vi "MP6_micro_pump.vi"() -> ()   [LabVIEW 2024]
uses:
  <vilib>/Instr/_visa.llb/VISA Configure Serial Port (Instr).vi
panel:
  out "P2V_output":string
  in  "P2V?":bool
  in  "Continuos V":bool
  out "P1V_output":string
  in  "P1V?":bool
  in  "P2V_value":u8
  in  "P2V_set":bool
  in  "F1_value":u8=100
  in  "F1_set":bool
  in  "P1V_value":u8=200
  in  "P1V_set":bool
  out "Output":string="150\r\n"
  in  "Input":string="P5V?\r\n"
  in  "Send Command":bool
  in  "P2OFF":bool
  in  "P2ON":bool
  in  "P1OFF":bool
  in  "P1ON":bool
  out "error out":errorcluster={"status"=FALSE, "code"=1073676294, "source"="VISA Read in MP6_micro_pump.vi"}
  in  "VISA resource name":refnum<visa-resource-name>="COM3"
  in  "Close connection":bool
  in  "Open connection":bool
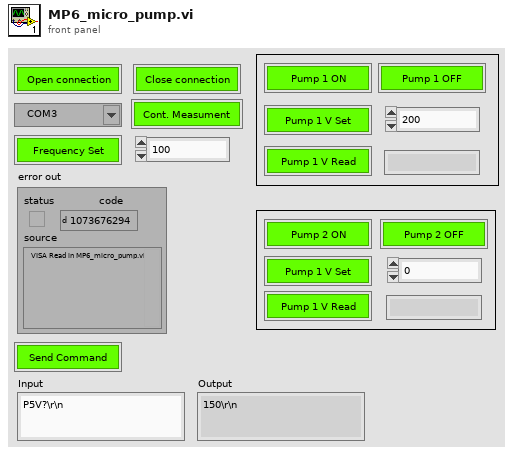
[diagram p1: front panel]
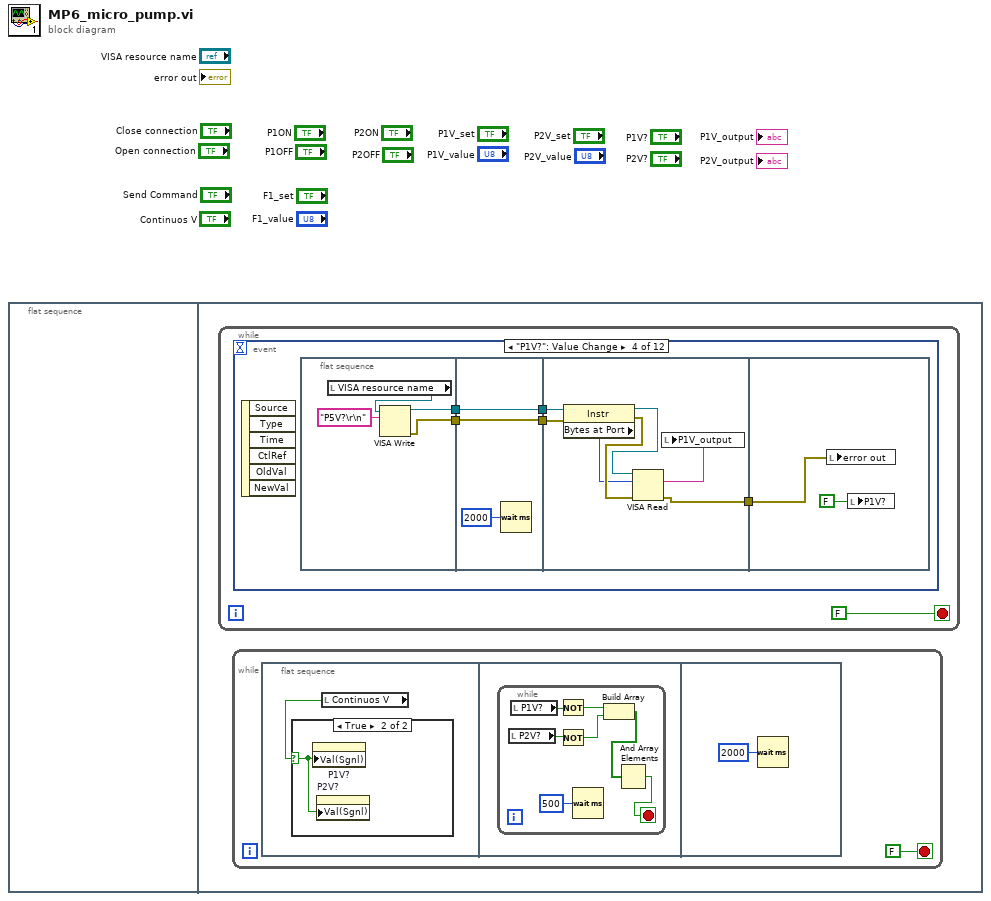
[diagram p0: block diagram]
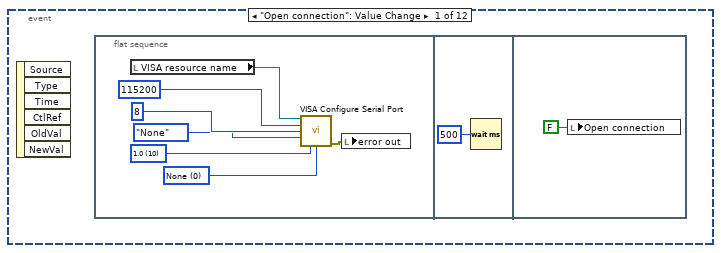
[diagram p3: hidden frame]
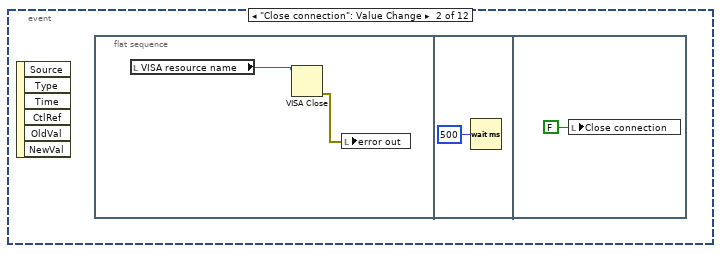
[diagram p4: hidden frame]
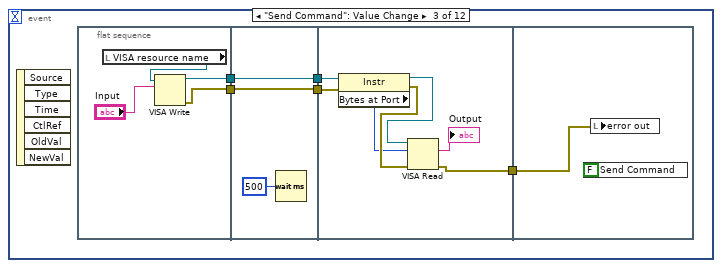
[diagram p5: hidden frame]
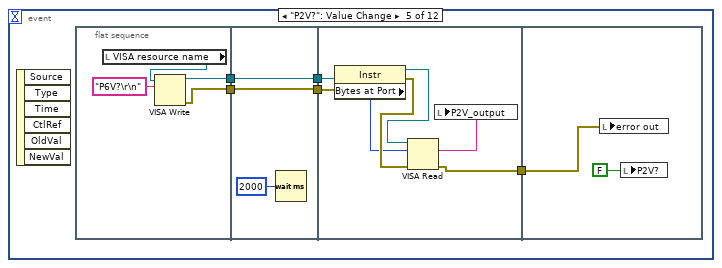
[diagram p6: hidden frame]
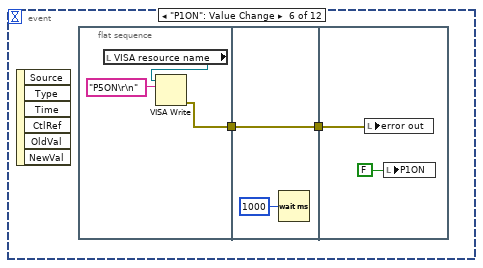
[diagram p7: hidden frame]
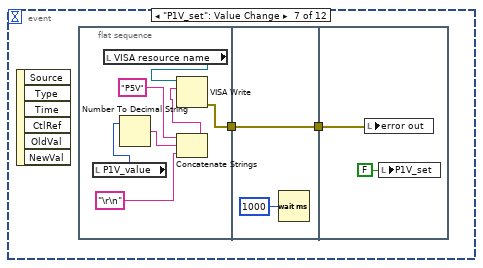
[diagram p8: hidden frame]
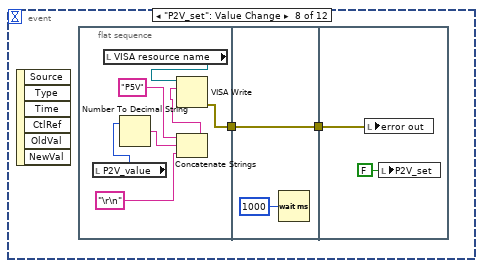
[diagram p9: hidden frame]
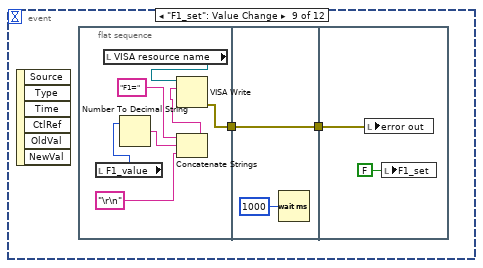
[diagram p10: hidden frame]
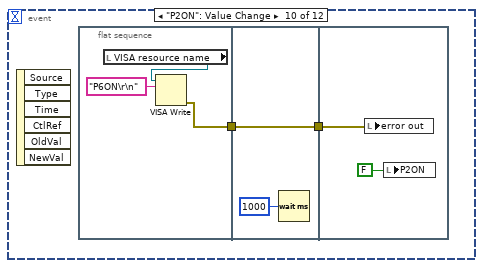
[diagram p11: hidden frame]
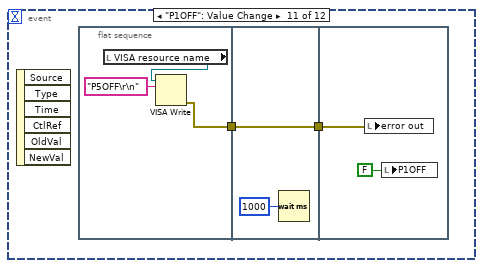
[diagram p12: hidden frame]
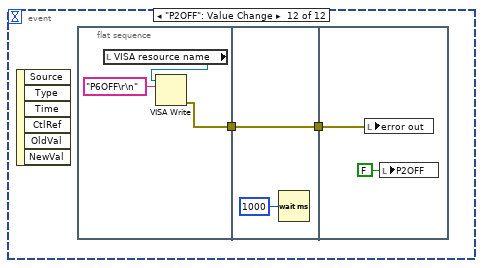
[diagram p13: hidden frame]
diagram:
  n1 = flat-sequence {
    frame #0 {
    }
    frame #1 {
      n2 = while {
        stop <- FALSE stop-if-true
        n3 = event shown="[3] \"P1V?\": Value Change" {
          selector: _ -> [_ _ _ _ _ _ _ _ _ _ _ _]
          dyn-events: _ -> [_ _ _ _ _ _ _ _ _ _ _ _]
          timeout: _ -> [_ _ _ _ _ _ _ _ _ _ _ _]
          event "Open connection": Value Change {
            n4 = event-data() -> ()  [unwired: 1 in, 6 out]
            n5 = flat-sequence {
              frame #0 {
                w15 = u16 0 items=["None", "XON/XOFF", "RTS/CTS", "XON/XOFF & RTS/CTS", "DTR/DSR", "XON/XOFF & DTR/DSR"] ("flow control (0:none)")
                w16 = u16 10 items=["1.0"=10, "1.5"=15, "2.0"=20] ("stop bits (10: 1 bit)")
                n6 = local read "VISA resource name"() -> (w13:refnum<visa-resource-name>)
                n7 = call-poly "VISA Configure Serial Port"("VISA resource name"=w13, "baud rate (9600)"=u32 115200, "data bits (8)"=u16 8, "parity (0:none)"=enum16{"None", "Odd", "Even", "Mark", "Space"}."None", "stop bits (10: 1 bit)"=w16, "flow control (0:none)"=w15) -> ("error out"=w14:errorcluster)  [unwired: 8 in, 1 out]
                n8 = local write "error out"(w14) -> ()
              }
              frame #1 {
                n9 = Wait (ms)(milliseconds to wait=u32 500) -> ()  [unwired: 1 out]
              }
              frame #2 {
                n10 = local write "Open connection"(FALSE ("Open connection")) -> ()
              }
            }
          }
          event "Close connection": Value Change {
            n11 = event-data() -> ()  [unwired: 1 in, 6 out]
            n12 = flat-sequence {
              frame #0 {
                n13 = local read "VISA resource name"() -> (w23:refnum<visa-resource-name>)
                n14 = VISA Close(VISA resource name=w23) -> (error out=w22:errorcluster)  [unwired: 1 in]
                n15 = local write "error out"(w22) -> ()
              }
              frame #1 {
                n16 = Wait (ms)(milliseconds to wait=u32 500) -> ()  [unwired: 1 out]
              }
              frame #2 {
                n17 = local write "Close connection"(FALSE ("Open connection")) -> ()
              }
            }
          }
          event "Send Command": Value Change {
            n18 = event-data() -> ()  [unwired: 1 in, 6 out]
            n19 = flat-sequence {
              tunnel: [w33] -> w29
              tunnel: [w31] -> w26
              tunnel: [w37] -> w30
              tunnel: w29 -> [w37]
              tunnel: [w36] -> w27
              tunnel: w26 -> [w36]
              tunnel: w30 -> [w43]
              tunnel: [w39] -> w28
              tunnel: w27 -> [w44]
              tunnel: w28 -> [w46]
              frame #0 {
                n20 = local read "VISA resource name"() -> (w34:refnum<visa-resource-name>)
                n21 = VISA Write(VISA resource name=w34, write buffer="Input") -> (VISA resource name out=w31:refnum<visa-resource-name>, error out=w33:errorcluster)  [unwired: 1 in, 1 out]
              }
              frame #1 {
                n22 = Wait (ms)(milliseconds to wait=u32 500) -> ()  [unwired: 1 out]
              }
              frame #2 {
                n23 = property class="Instr"(reference=w44, error in=w43) -> (reference out=w41:refnum<visa-resource-name>, error out=w42:errorcluster, "Bytes at Port"=w40:u32)
                n24 = VISA Read(VISA resource name=w41, byte count=w40, error in (no error)=w42) -> (read buffer=→"Output":string, error out=w39:errorcluster)  [unwired: 2 out]
              }
              frame #3 {
                n25 = local write "Send Command"(FALSE ("P1OFF")) -> ()
                n26 = local write "error out"(w46) -> ()
              }
            }
          }
          event "P1V?": Value Change {
            n27 = event-data() -> ()  [unwired: 1 in, 6 out]
            n28 = flat-sequence {
              tunnel: [w54] -> w50
              tunnel: [w53] -> w47
              tunnel: [w58] -> w51
              tunnel: w50 -> [w58]
              tunnel: [w57] -> w48
              tunnel: w47 -> [w57]
              tunnel: w51 -> [w64]
              tunnel: [w60] -> w49
              tunnel: w48 -> [w65]
              tunnel: w49 -> [w67]
              frame #0 {
                n29 = local read "VISA resource name"() -> (w55:refnum<visa-resource-name>)
                n30 = VISA Write(VISA resource name=w55, write buffer="P5V?\r\n") -> (VISA resource name out=w53:refnum<visa-resource-name>, error out=w54:errorcluster)  [unwired: 1 in, 1 out]
              }
              frame #1 {
                n31 = Wait (ms)(milliseconds to wait=u32 2000) -> ()  [unwired: 1 out]
              }
              frame #2 {
                n32 = property class="Instr"(reference=w65, error in=w64) -> (reference out=w62:refnum<visa-resource-name>, error out=w63:errorcluster, "Bytes at Port"=w61:u32)
                n33 = VISA Read(VISA resource name=w62, byte count=w61, error in (no error)=w63) -> (read buffer=w59:string, error out=w60:errorcluster)  [unwired: 2 out]
                n34 = local write "P1V_output"(w59) -> ()
              }
              frame #3 {
                n35 = local write "error out"(w67) -> ()
                n36 = local write "P1V?"(FALSE ("P1OFF")) -> ()
              }
            }
          }
          event "P2V?": Value Change {
            n37 = event-data() -> ()  [unwired: 1 in, 6 out]
            n38 = flat-sequence {
              tunnel: [w75] -> w71
              tunnel: [w74] -> w68
              tunnel: [w79] -> w72
              tunnel: w71 -> [w79]
              tunnel: [w78] -> w69
              tunnel: w68 -> [w78]
              tunnel: w72 -> [w85]
              tunnel: [w81] -> w70
              tunnel: w69 -> [w86]
              tunnel: w70 -> [w88]
              frame #0 {
                n39 = local read "VISA resource name"() -> (w76:refnum<visa-resource-name>)
                n40 = VISA Write(VISA resource name=w76, write buffer="P6V?\r\n") -> (VISA resource name out=w74:refnum<visa-resource-name>, error out=w75:errorcluster)  [unwired: 1 in, 1 out]
              }
              frame #1 {
                n41 = Wait (ms)(milliseconds to wait=u32 2000) -> ()  [unwired: 1 out]
              }
              frame #2 {
                n42 = property class="Instr"(reference=w86, error in=w85) -> (reference out=w83:refnum<visa-resource-name>, error out=w84:errorcluster, "Bytes at Port"=w82:u32)
                n43 = VISA Read(VISA resource name=w83, byte count=w82, error in (no error)=w84) -> (read buffer=w80:string, error out=w81:errorcluster)  [unwired: 2 out]
                n44 = local write "P2V_output"(w80) -> ()
              }
              frame #3 {
                n45 = local write "error out"(w88) -> ()
                n46 = local write "P2V?"(FALSE ("P1OFF")) -> ()
              }
            }
          }
          event "P1ON": Value Change {
            n47 = event-data() -> ()  [unwired: 1 in, 6 out]
            n48 = flat-sequence {
              tunnel: [w91] -> w89
              tunnel: [w94] -> w90
              tunnel: w89 -> [w94]
              tunnel: w90 -> [w96]
              frame #0 {
                n49 = local read "VISA resource name"() -> (w93:refnum<visa-resource-name>)
                n50 = VISA Write(VISA resource name=w93, write buffer="P5ON\r\n") -> (error out=w91:errorcluster)  [unwired: 1 in, 2 out]
              }
              frame #1 {
                n51 = Wait (ms)(milliseconds to wait=u32 1000) -> ()  [unwired: 1 out]
              }
              frame #2 {
                n52 = local write "error out"(w96) -> ()
                n53 = local write "P1ON"(FALSE ("P1OFF")) -> ()
              }
            }
          }
          event "P1V_set": Value Change {
            n54 = event-data() -> ()  [unwired: 1 in, 6 out]
            n55 = flat-sequence {
              tunnel: [w105] -> w98
              tunnel: [w107] -> w99
              tunnel: w98 -> [w107]
              tunnel: w99 -> [w109]
              frame #0 {
                n56 = local read "P1V_value"() -> (w104:u8)
                n57 = local read "VISA resource name"() -> (w106:refnum<visa-resource-name>)
                n58 = Number To Decimal String(number=w104) -> (decimal integer string=w103:string)  [unwired: 1 in]
                n59 = Concatenate Strings("P5V" ("write buffer"), w103, "\r\n" ("write buffer")) -> (w100:string)
                n60 = VISA Write(VISA resource name=w106, write buffer=w100) -> (error out=w105:errorcluster)  [unwired: 1 in, 2 out]
              }
              frame #1 {
                n61 = Wait (ms)(milliseconds to wait=u32 1000) -> ()  [unwired: 1 out]
              }
              frame #2 {
                n62 = local write "error out"(w109) -> ()
                n63 = local write "P1V_set"(FALSE ("P1OFF")) -> ()
              }
            }
          }
          event "P2V_set": Value Change {
            n64 = event-data() -> ()  [unwired: 1 in, 6 out]
            n65 = flat-sequence {
              tunnel: [w118] -> w111
              tunnel: [w120] -> w112
              tunnel: w111 -> [w120]
              tunnel: w112 -> [w122]
              frame #0 {
                n66 = local read "P2V_value"() -> (w117:u8)
                n67 = local read "VISA resource name"() -> (w119:refnum<visa-resource-name>)
                n68 = Number To Decimal String(number=w117) -> (decimal integer string=w116:string)  [unwired: 1 in]
                n69 = Concatenate Strings("P5V" ("write buffer"), w116, "\r\n" ("write buffer")) -> (w113:string)
                n70 = VISA Write(VISA resource name=w119, write buffer=w113) -> (error out=w118:errorcluster)  [unwired: 1 in, 2 out]
              }
              frame #1 {
                n71 = Wait (ms)(milliseconds to wait=u32 1000) -> ()  [unwired: 1 out]
              }
              frame #2 {
                n72 = local write "error out"(w122) -> ()
                n73 = local write "P2V_set"(FALSE ("P1OFF")) -> ()
              }
            }
          }
          event "F1_set": Value Change {
            n74 = event-data() -> ()  [unwired: 1 in, 6 out]
            n75 = flat-sequence {
              tunnel: [w131] -> w124
              tunnel: [w133] -> w125
              tunnel: w124 -> [w133]
              tunnel: w125 -> [w135]
              frame #0 {
                n76 = local read "F1_value"() -> (w130:u8)
                n77 = local read "VISA resource name"() -> (w132:refnum<visa-resource-name>)
                n78 = Number To Decimal String(number=w130) -> (decimal integer string=w129:string)  [unwired: 1 in]
                n79 = Concatenate Strings("F1=" ("write buffer"), w129, "\r\n" ("write buffer")) -> (w126:string)
                n80 = VISA Write(VISA resource name=w132, write buffer=w126) -> (error out=w131:errorcluster)  [unwired: 1 in, 2 out]
              }
              frame #1 {
                n81 = Wait (ms)(milliseconds to wait=u32 1000) -> ()  [unwired: 1 out]
              }
              frame #2 {
                n82 = local write "error out"(w135) -> ()
                n83 = local write "F1_set"(FALSE ("P1OFF")) -> ()
              }
            }
          }
          event "P2ON": Value Change {
            n84 = event-data() -> ()  [unwired: 1 in, 6 out]
            n85 = flat-sequence {
              tunnel: [w139] -> w137
              tunnel: [w142] -> w138
              tunnel: w137 -> [w142]
              tunnel: w138 -> [w144]
              frame #0 {
                n86 = local read "VISA resource name"() -> (w141:refnum<visa-resource-name>)
                n87 = VISA Write(VISA resource name=w141, write buffer="P6ON\r\n") -> (error out=w139:errorcluster)  [unwired: 1 in, 2 out]
              }
              frame #1 {
                n88 = Wait (ms)(milliseconds to wait=u32 1000) -> ()  [unwired: 1 out]
              }
              frame #2 {
                n89 = local write "error out"(w144) -> ()
                n90 = local write "P2ON"(FALSE ("P1OFF")) -> ()
              }
            }
          }
          event "P1OFF": Value Change {
            n91 = event-data() -> ()  [unwired: 1 in, 6 out]
            n92 = flat-sequence {
              tunnel: [w148] -> w146
              tunnel: [w151] -> w147
              tunnel: w146 -> [w151]
              tunnel: w147 -> [w153]
              frame #0 {
                n93 = local read "VISA resource name"() -> (w150:refnum<visa-resource-name>)
                n94 = VISA Write(VISA resource name=w150, write buffer="P5OFF\r\n") -> (error out=w148:errorcluster)  [unwired: 1 in, 2 out]
              }
              frame #1 {
                n95 = Wait (ms)(milliseconds to wait=u32 1000) -> ()  [unwired: 1 out]
              }
              frame #2 {
                n96 = local write "error out"(w153) -> ()
                n97 = local write "P1OFF"(FALSE ("P1OFF")) -> ()
              }
            }
          }
          event "P2OFF": Value Change {
            n98 = event-data() -> ()  [unwired: 1 in, 6 out]
            n99 = flat-sequence {
              tunnel: [w157] -> w155
              tunnel: [w160] -> w156
              tunnel: w155 -> [w160]
              tunnel: w156 -> [w162]
              frame #0 {
                n100 = local read "VISA resource name"() -> (w159:refnum<visa-resource-name>)
                n101 = VISA Write(VISA resource name=w159, write buffer="P6OFF\r\n") -> (error out=w157:errorcluster)  [unwired: 1 in, 2 out]
              }
              frame #1 {
                n102 = Wait (ms)(milliseconds to wait=u32 1000) -> ()  [unwired: 1 out]
              }
              frame #2 {
                n103 = local write "error out"(w162) -> ()
                n104 = local write "P2OFF"(FALSE ("P1OFF")) -> ()
              }
            }
          }
        }
      }
      n105 = while {
        stop <- FALSE stop-if-true
        n106 = flat-sequence {
          frame #0 {
            n107 = local read "Continuos V"() -> (w2:bool)
            n108 = case shown="True" w2 {
              selector: w2 -> [_ w3]
              frame False {
              }
              frame True {
                n109 = property on="P1V?" class="Bool (strict)"("Val(Sgnl)"=w3) -> ()  [unwired: 2 in, 2 out]
                n110 = property on="P2V?" class="Bool (strict)"("Val(Sgnl)"=w3) -> ()  [unwired: 2 in, 2 out]
              }
            }
          }
          frame #1 {
            n111 = while {
              stop <- w8 stop-if-true
              n112 = local read "P2V?"() -> (w5:bool)
              n113 = local read "P1V?"() -> (w10:bool)
              n114 = Not(x=w10) -> (.not. x?=w9:bool)
              n115 = Not(x=w5) -> (.not. x?=w4:bool)
              n116 = Wait (ms)(milliseconds to wait=u32 500) -> ()  [unwired: 1 out]
              n117 = Build Array(w9, w4) -> (w7:bool[])
              n118 = And Array Elements(Boolean array=w7) -> (logical AND=w8:bool)
            }
          }
          frame #2 {
            n119 = Wait (ms)(milliseconds to wait=u32 2000) -> ()  [unwired: 1 out]
          }
        }
      }
    }
  }
